vi "Read add enable channel.vi"(8 "error in (no error)":errorcluster, 11 "bin datalogger configuration in":refnum<class "Binary datalogger configuration.lvclass">) -> (0 "error out":errorcluster, 2 "add enable channel":bool, 3 "bin datalogger configuration out":refnum<class "Binary datalogger configuration.lvclass">)   [LabVIEW 2013, in "Binary datalogger configuration.lvclass"]
uses:
  Binary datalogger configuration.lvclass
  Binary datalogger configuration.lvclass/Binary datalogger configuration.ctl
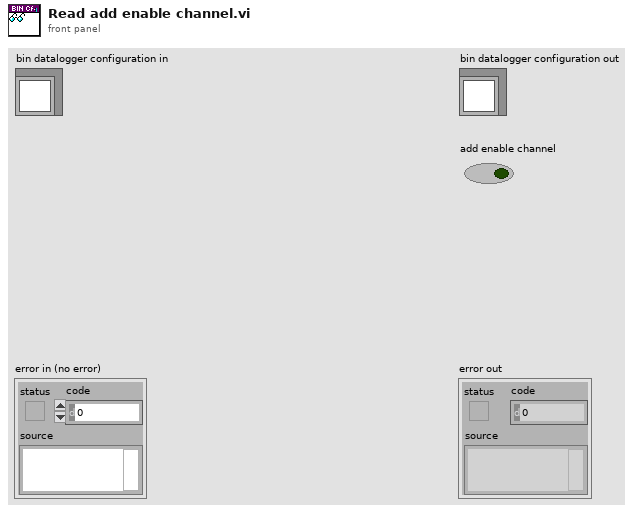
[diagram p1: front panel]
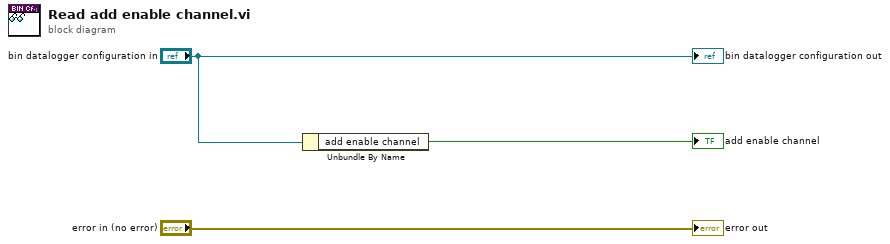
[diagram p0: block diagram]
diagram:
  n1 = Unbundle By Name("bin datalogger configuration in") -> ("add enable channel"=→"add enable channel":bool)
  "error out" <- "error in (no error)"
  "bin datalogger configuration out" <- "bin datalogger configuration in"
